vi "SetServoState.vi"(8 "Servo State":i32, 10 "Controller Channel":i32, 11 "Handle":u32) -> (3 "FT_Status":u32(ring) items=["FT_OK", "FT_INVALID_HANDLE", "FT_DEVICE_NOT_FOUND", "FT_DEVICE_NOT_OPENED", "FT_IO_ERROR", "FT_INSUFFICIENT_RESOURCES", "FT_INVALID_PARAMETER", "FT_INVALID_BAUD_RATE", "FT_DEVICE_NOT_OPENED_FOR_ERASE", "FT_DEVICE_NOT_OPENED_FOR_WRITE", "FT_FAILED_TO_WRITE_DEVICE", "FT_EEPROM_READ_FAILED", "FT_EEPROM_WRITE_FAILED", "FT_EEPROM_ERASE_FAILED", "FT_EEPROM_NOT_PRESENT", "FT_EEPROM_NOT_PROGRAMMED", "FT_INVALID_ARGS", "FT_NOT_SUPPORTED", "FT_OTHER_ERROR"])   [LabVIEW 2011]
panel:
  out "Bytes Written":u32
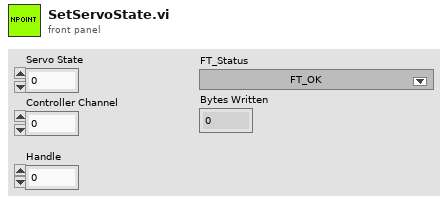
[diagram p1: front panel]
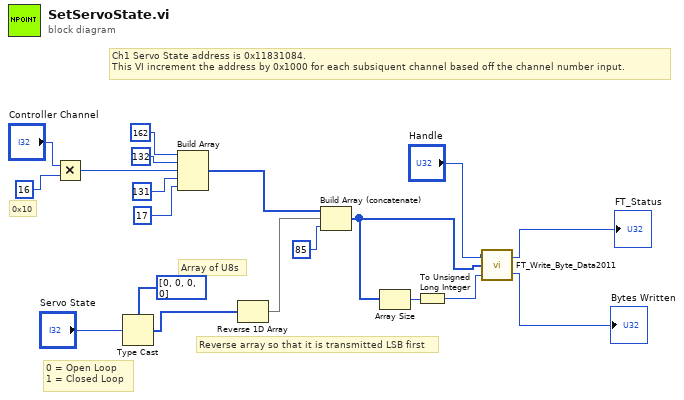
[diagram p0: block diagram]
diagram:
  # "0 = Open Loop\n1 = Closed Loop"
  # "Reverse array so that it is transmitted LSB first"
  # "Ch1 Servo State address is 0x11831084.\nThis VI increment the address by 0x1000 for each subsiquent channel based off the channel number input."
  # "0x10"
  # "Array of U8s"
  n1 = Multiply(x="Controller Channel", y=u8 16) -> (x*y=w6:i32)
  n2 = Type Cast(type=u8[] [0, 0, 0, 0], x="Servo State") -> (*(type *) &x=w11:u8[])
  n3 = Build Array(u8 162 ("element"), u8 132 ("element"), w6, u8 131 ("element"), u8 17 ("element")) -> (w13:i32[])
  n4 = Reverse 1D Array(array=w11) -> (reversed array=w10:u8[])
  n5 = Build Array (concatenate)(w13, w10, u8 85 ("element")) -> (w4:i32[])
  n6 = Array Size(array=w4) -> (size(s)=w19:i32)
  n7 = To Unsigned Long Integer(number=w19) -> (unsigned 32bit integer=w3:u32)
  n8 = call "FT_Write_Byte_Data2011.vi"("Bytes To Write"=w3, "Buffer"=w4, "Handle"="Handle") -> ("Bytes Written"=→"Bytes Written":u32, "FT_Status"=→"FT_Status":u32)
